vi "LvDatatypeToImageType_2DArray-SGL.vi"(9 "error in":errorcluster, 11 "Array":sgl[][](array[numeric])) -> (1 "error out":errorcluster, 2 "Image Type":T1, 3 "Array out":sgl[][](array[numeric]))   [LabVIEW 2020, in "OpenLvVision_OpenCv.lvlib"]
doc: "converts 2d array to image format"
uses:
  OpenLvVision_OpenCv.lvlib
  <vilib>/OpenLvVision/OpenLvVision_Image/Management/TypeDef/OLV ImageType.ctl
  <vilib>/OpenLvVision/OpenLvVision_Image/Management/OLV Management.lvlib
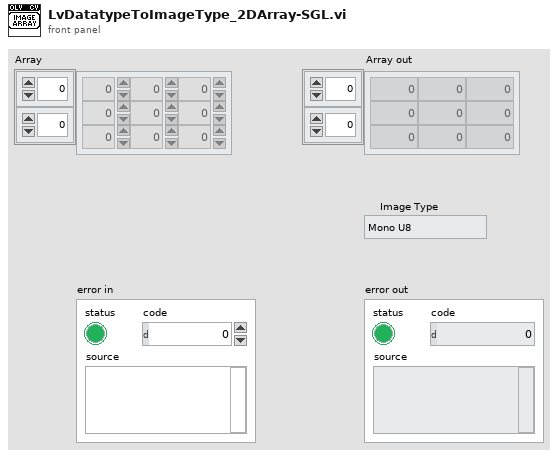
[diagram p1: front panel]
types:
  T1 = typedef "OLV OpenLvVision_Image.lvlib/OLV Management.lvlib/OLV ImageType.ctl" = enum16{"Mono U8", "Mono U16", "Mono I16", "Mono SGL", "Color U32", "Color U64", "Complex CSG"}
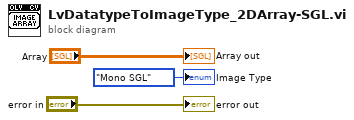
[diagram p0: block diagram]
diagram:
  "Array out" <- "Array"
  "Image Type" <- OLV_ImageType."Mono SGL" ("Image Type")
  "error out" <- "error in"
